vi "ADC Read.vi"(10 "DataNum":i32, 11 "DevIndex":i32) -> (2 "function return":i32, 3 "pData":i16[](array[numeric]))   [LabVIEW 2010, in "usb2adc.lvlib"]
doc: "int WINAPI ADC_Read(int DevIndex,short *pData,int DataNum);"
uses:
  usb2adc.lvlib
  USB2XXX.dll
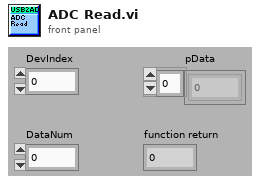
[diagram p1: front panel]
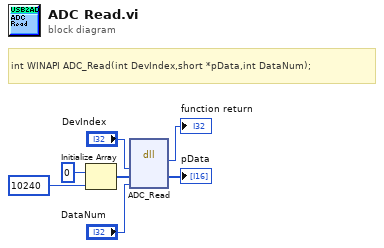
[diagram p0: block diagram]
diagram:
  # "int WINAPI ADC_Read(int DevIndex,short *pData,int DataNum);"
  n1 = Initialize Array(i16 0 ("element"), 10240 ("dimension size")) -> (w5:i16[])
  n2 = dll-call lib="G:/OtherWork/USB2XXX_Example/trunk/Labview/PublicFiles/usb2adc/USB2XXX.*" fn="ADC_Read"("DevIndex"="DevIndex", "pData"=w5, "DataNum"="DataNum") -> (→"function return":i32, "pData"=→"pData":i16[])  [unwired: 5 in, 2 out]
